vi "Example Main Program.vi"() -> ()   [LabVIEW 2018]
uses:
  <vilib>/Platform/TimedLoop/XDataNode/timing_clust.ctl
  <vilib>/Platform/TimedLoop/XDataNode/nitl_modes.ctl
  <vilib>/Platform/TimedLoop/XDataNode/wakeup.ctl
  <vilib>/platform/TimedLoop/XDataNode/XDataNode.xnode
  <vilib>/Platform/TimedLoop/XDataNode/XDNodeRunTimeDep.lvlib
  COBRA Prosthesis Model Library.lvlib
  <vilib>/ptbypt/NI_PtbyPt.lvlib
panel:
  out "Prosthesis Angle (deg)":dbl(graph)
  out "Joint Torque Setpoint (Nm)":dbl(graph)
  in  "Stop":bool
  out "Cable Force Setpoint (N)":dbl(graph)
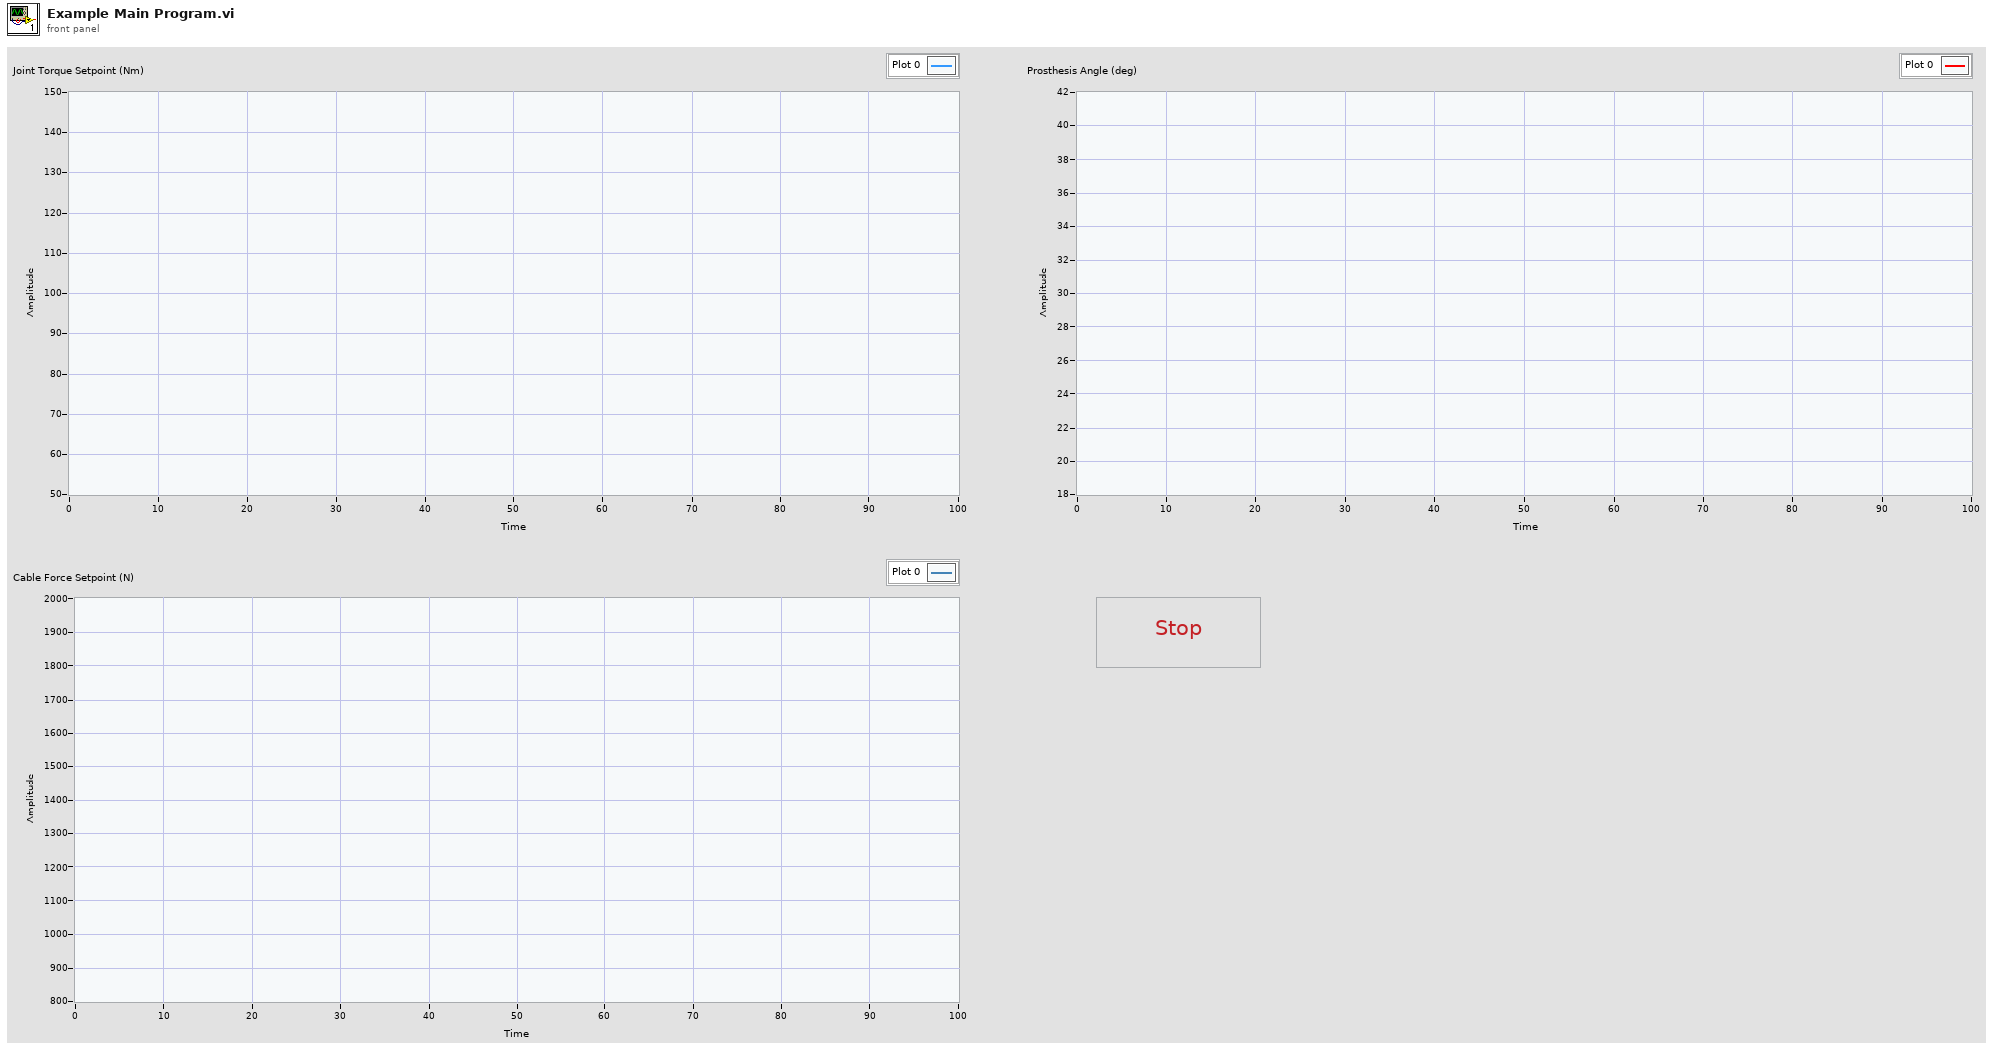
[diagram p1: front panel]
types:
  T1 = typedef "XDNodeRunTimeDep.lvlib/timing_clust.ctl" = cluster{"Expected End [f-1]":u64, "Actual End [f-1]":u64, "Finished Late? [f-1]":bool, "Expected End [i-1]":u64, "Actual End [i-1]":u64, "Finished Late? [i-1]":bool, "Expected Start [i]":u64, "Actual Start [i]":u64, "Expected Start [f]":u64, "Actual Start [f]":u64, "Source Name":string, "Structure Name":string, "Period":i64, "Deadline":i64, "Offset":i64, "Start":i64, "Priority":i32, "Timeout":i32, "Mode":T2, "Wakeup Reason":T3, "Error":errorcluster, "Source Type":string, "Secondary Source Type":string, "Global End Time":u64, "Global Start Time":u64, "Frame Duration":u64, "Iteration Duration":u64, "Assigned CPU":i32, "I/O Scan Engine Mode":u32}
  T2 = typedef "XDNodeRunTimeDep.lvlib/nitl_modes.ctl" = enum32{"No Change", "Process missed periods, maintain original phase", "Discard missed periods, maintain original phase", "Process missed periods, ignore original phase", "Discard missed periods, ignore original phase"}
  T3 = typedef "XDNodeRunTimeDep.lvlib/wakeup.ctl" = enum32{"Normal", "Aborted", "Asynchronous wakeup", "Timing source error", "Timed loop error", "Timeout"}
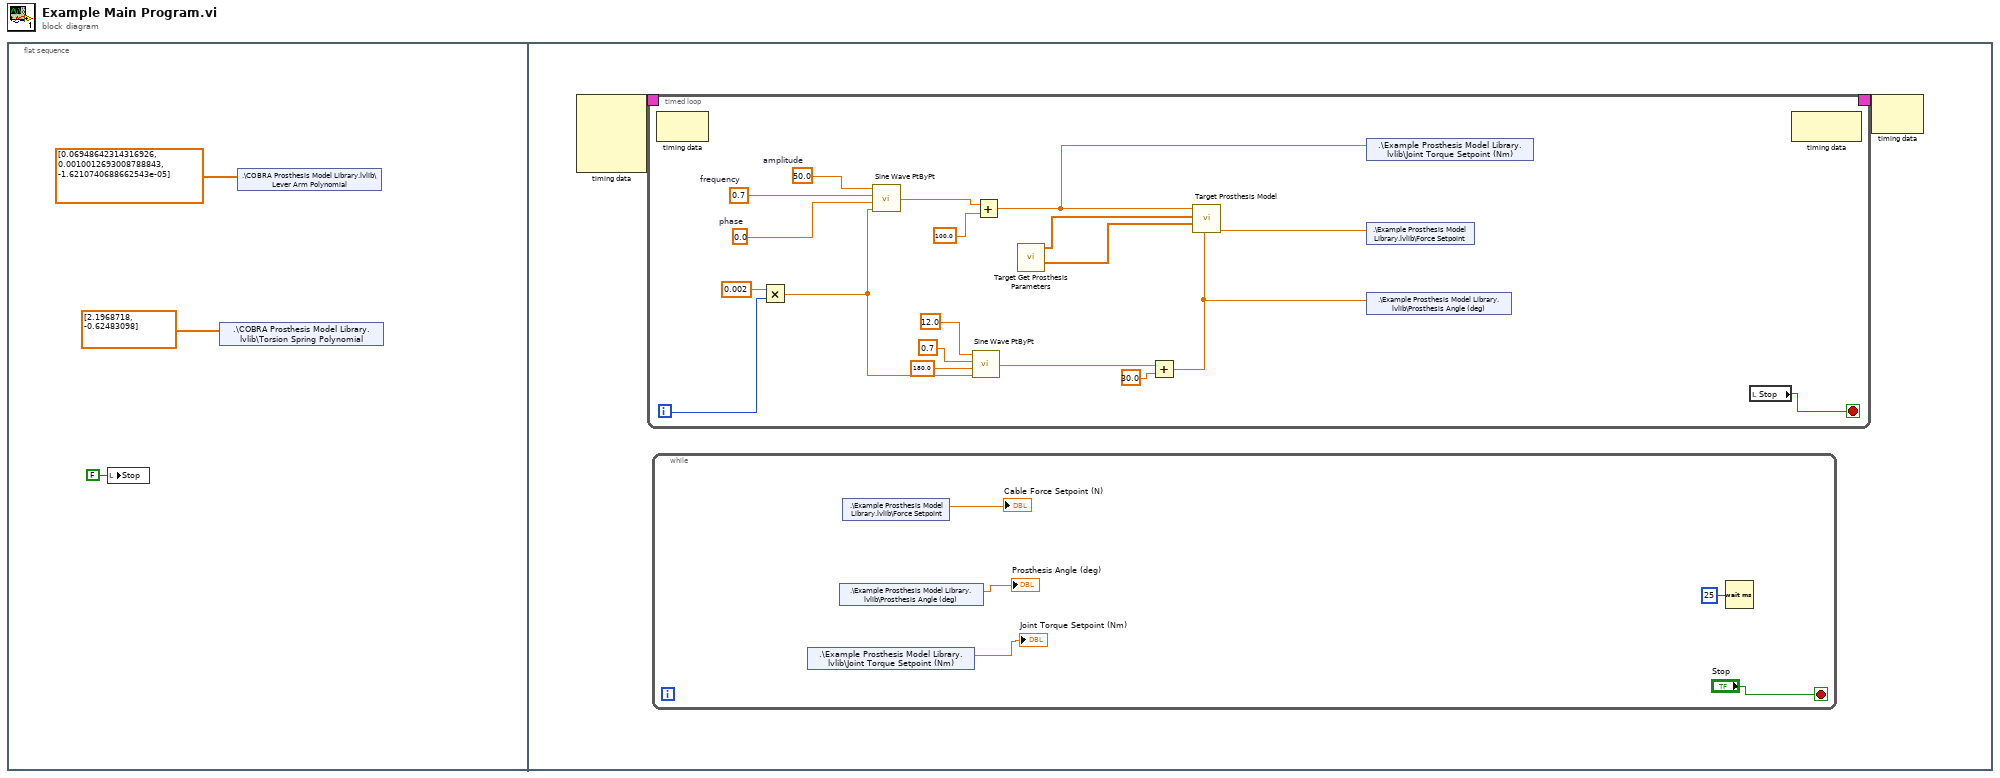
[diagram p0: block diagram]
diagram:
  n1 = flat-sequence {
    frame #0 {
      n2 = local write "Stop"(FALSE ("Stop")) -> ()
      n3 = shared-variable ".\\COBRA Prosthesis Model Library.lvlib\\Torsion Spring Polynomial"(dbl[] [2.1968718, -0.62483098] ("P(x)")) -> ()  [unwired: 1 in, 1 out]
      n4 = shared-variable ".\\COBRA Prosthesis Model Library.lvlib\\Lever Arm Polynomial"(dbl[] [0.06948642314316926, 0.0010012693008788843, -1.6210740688662543e-05] ("P(x)")) -> ()  [unwired: 1 in, 1 out]
    }
    frame #1 {
      n5 = node-c288() -> (w5:T1)  [unwired: 4 in]
      n6 = timed-loop {
        timing: w5 -> [_]
        timing-out: [_] -> w4
        i -> [w25]
        stop <- w20 stop-if-true
        w27 = 0.0  # phase
        w28 = 0.7  # frequency
        w29 = 50.0  # amplitude
        n7 = node-c288() -> ()  [unwired: 1 in, 1 out]
        n8 = Multiply(x=0.002, y=w25) -> (x*y=w19:dbl)
        n9 = call <vilib>:"Sine Wave PtByPt.vi"("time"=w19, "phase"=w27, "frequency"=w28, "amplitude"=w29) -> ("sine wave"=w15:dbl)
        n10 = call <vilib>:"Sine Wave PtByPt.vi"("time"=w19, "phase"=180.0, "frequency"=0.7, "amplitude"=12.0) -> ("sine wave"=w13:dbl)
        n11 = Add(x=w15, y=100.0) -> (x+y=w14:dbl)
        n12 = call "Target Get Prosthesis Parameters.vi"() -> ("Lever Arm Polynomial"=w22:dbl[], "Spring Polynomial"=w23:dbl[])  [unwired: 10 in]
        n13 = Add(x=w13, y=30.0) -> (x+y=w11:dbl)
        n14 = call "Target Prosthesis Model.vi"("Prosthesis Angle (degrees)"=w11, "Lever Arm Polynomial"=w22, "Spring Polynomial"=w23, "Joint Torque Setpoint (Nm)"=w14) -> ("Force Setpoint (N)"=w21:dbl)  [unwired: 7 in]
        n15 = shared-variable ".\\Example Prosthesis Model Library.lvlib\\Joint Torque Setpoint (Nm)"(w14) -> ()  [unwired: 1 in, 1 out]
        n16 = shared-variable ".\\Example Prosthesis Model Library.lvlib\\Force Setpoint"(w21) -> ()  [unwired: 1 in, 1 out]
        n17 = shared-variable ".\\Example Prosthesis Model Library.lvlib\\Prosthesis Angle (deg)"(w11) -> ()  [unwired: 1 in, 1 out]
        n18 = local read "Stop"() -> (w20:bool)
        n19 = node-c288() -> ()  [unwired: 1 in, 1 out]
      }
      n20 = while {
        stop <- "Stop" stop-if-true
        n21 = shared-variable ".\\Example Prosthesis Model Library.lvlib\\Joint Torque Setpoint (Nm)"() -> (→"Joint Torque Setpoint (Nm)":dbl)  [unwired: 1 in, 1 out]
        n22 = shared-variable ".\\Example Prosthesis Model Library.lvlib\\Prosthesis Angle (deg)"() -> (→"Prosthesis Angle (deg)":dbl)  [unwired: 1 in, 1 out]
        n23 = shared-variable ".\\Example Prosthesis Model Library.lvlib\\Force Setpoint"() -> (→"Cable Force Setpoint (N)":dbl)  [unwired: 1 in, 1 out]
        n24 = Wait (ms)(milliseconds to wait=u32 25) -> ()  [unwired: 1 out]
      }
      n25 = node-c288(w4) -> ()  [unwired: 1 out]
    }
  }
